vi "U8翻转.vi"(1 "x":u8) -> (0 "z":u8)   [LabVIEW 2012]
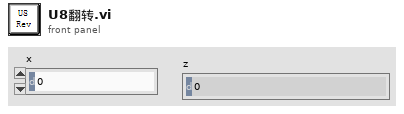
[diagram p1: front panel]
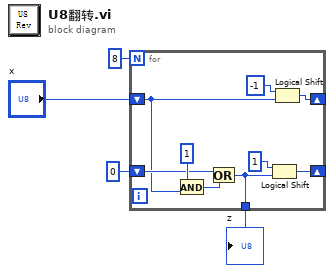
[diagram p0: block diagram]
diagram:
  n1 = for {
    N: 8 -> [_]
    shift-right: [w12] -> _
    shift-left: "x" -> [w6]
    shift-right: [w9] -> _
    shift-left: u8 0 ("x") -> [w7]
    tunnel: [w5] -> w1
    n2 = And(x=u8 1, y=w6) -> (x .and. y?=w8:u8)
    n3 = Or(x=w7, y=w8) -> (x .or. y?=w5:u8)
    n4 = Logical Shift(y=i16 1, x=w5) -> (x << y=w9:u8)
    n5 = Logical Shift(y=i16 -1, x=w6) -> (x << y=w12:u8)
  }
  "z" <- w1
